vi "MCS_Backlash Test.vi"() -> ()   [LabVIEW 2010]
uses:
  <vilib>/Utility/file.llb/Write To Spreadsheet File (DBL).vi
panel:
  out "Current Round":i32
  out "Position (um)":dbl
  in  "Save File Name":string
  in  "Path":path
  in  "Moving Distance (um)":dbl
  in  "Channel":u32
  in  "Number of Round":i32
  in  "MCS System Locator":string
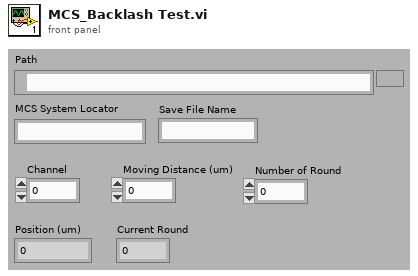
[diagram p1: front panel]
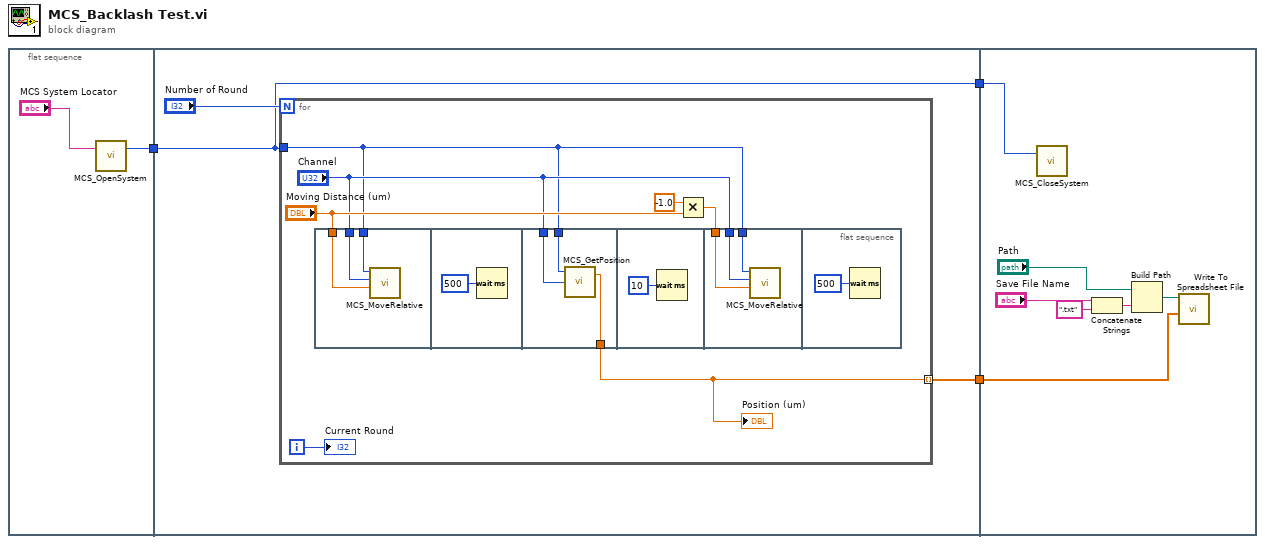
[diagram p0: block diagram]
diagram:
  n1 = flat-sequence {
    tunnel: [w4] -> w3
    tunnel: w3 -> [w7]
    tunnel: [w7] -> w2
    tunnel: [w6] -> w1
    tunnel: w2 -> [w34]
    tunnel: w1 -> [w28]
    frame #0 {
      n2 = call "MCS_OpenSystem.vi"("MCS System Locator"="MCS System Locator") -> ("System Index Out"=w4:u32)  [unwired: 1 in, 1 out]
    }
    frame #1 {
      n3 = for {
        N: "Number of Round" -> [_]
        tunnel: w7 -> [w9]
        tunnel: [w13] -> w6 mode=indexing
        i -> [w12]
        n4 = flat-sequence {
          tunnel: w9 -> [w18]
          tunnel: "Channel" -> [w17]
          tunnel: "Moving Distance (um)" -> [w16]
          tunnel: w9 -> [w22]
          tunnel: "Channel" -> [w21]
          tunnel: [w20] -> w13
          tunnel: w14 -> [w26]
          tunnel: "Channel" -> [w25]
          tunnel: w9 -> [w24]
          frame #0 {
            n5 = call "MCS_MoveRelative.vi"("Moving Distance (um)"=w16, "Channel Index In"=w17, "System Index In"=w18) -> ()  [unwired: 1 in, 1 out]
          }
          frame #1 {
            n6 = Wait (ms)(milliseconds to wait=u32 500) -> ()  [unwired: 1 out]
          }
          frame #2 {
            n7 = call "MCS_GetPosition.vi"("Channel Index In"=w21, "System Index In"=w22) -> ("Position (um)"=w20:dbl)  [unwired: 1 in, 1 out]
          }
          frame #3 {
            n8 = Wait (ms)(milliseconds to wait=u32 10) -> ()  [unwired: 1 out]
          }
          frame #4 {
            n9 = call "MCS_MoveRelative.vi"("Moving Distance (um)"=w26, "Channel Index In"=w25, "System Index In"=w24) -> ()  [unwired: 1 in, 1 out]
          }
          frame #5 {
            n10 = Wait (ms)(milliseconds to wait=u32 500) -> ()  [unwired: 1 out]
          }
        }
        n11 = Multiply(x=-1.0, y="Moving Distance (um)") -> (x*y=w14:dbl)
        "Position (um)" <- w13
        "Current Round" <- w12
      }
    }
    frame #2 {
      n12 = call "MCS_CloseSystem.vi"("System Index In"=w34) -> ()  [unwired: 1 in, 1 out]
      n13 = Concatenate Strings("Save File Name", ".txt" ("string")) -> (w32:string)
      n14 = Build Path(base path="Path", name or relative path=w32) -> (appended path=w33:path)
      n15 = call-poly <vilib>:"Write To Spreadsheet File.vi"("1D data"=w28, "file path (dialog if empty)"=w33) -> ()  [unwired: 6 in, 1 out]
    }
  }
